vi "UpdateArrayHeightWidth.vi"(7 "Borders in Percent(T) or Pixels (F)":bool, 8 "error in (no error)":errorcluster, 9 "Adjust":u16(ring) items=["Height", "Width", "Both"], 10 "Borders":T1, 11 "Array in":refnum<vi>) -> (0 "error out":errorcluster)   [LabVIEW 2022 SP3, in "PentaPanesLibrary.lvlib" / "PentaPanes.lvclass"]
uses:
  PentaPanes.lvclass
  BordersCluster.ctl
  <vilib>/Utility/miscctls.llb/LVPositionTypeDef.ctl
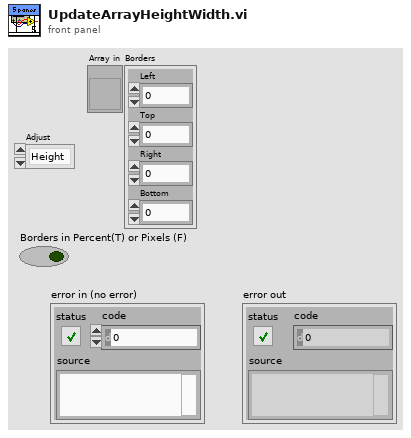
[diagram p1: front panel]
types:
  T1 = typedef "PentaPanesLibrary.lvlib/PentaPanes.lvclass/BordersCluster.ctl" = cluster{"Left":i32, "Top":i32, "Right":i32, "Bottom":i32}
  T2 = typedef "LVPositionTypeDef.ctl" = cluster{"Left":i32, "Top":i32}
  T3 = typedef "LVBoundsTypeDef.ctl" = cluster{"Width":u32, "Height":u32}
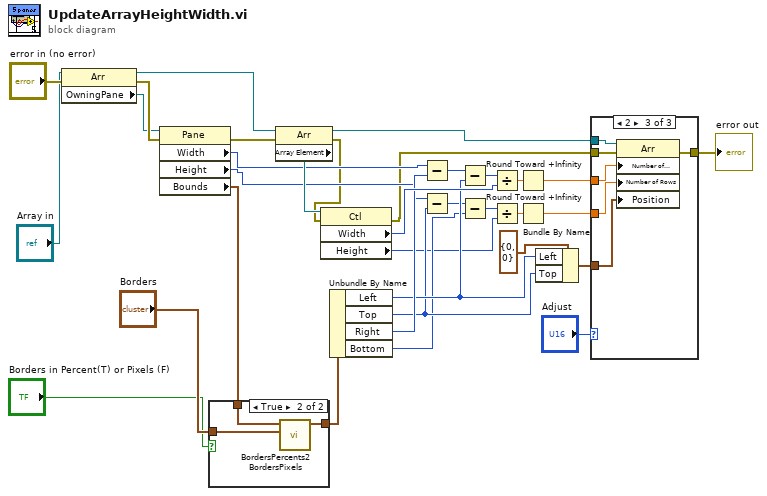
[diagram p0: block diagram]
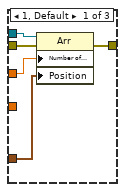
[diagram p3: hidden frame]
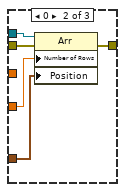
[diagram p4: hidden frame]
diagram:
  n1 = property class="Arr"(reference="Array in", error in="error in (no error)") -> (reference out=w3:refnum<vi>, error out=w33:errorcluster, "OwningPane"=w31:refnum<vi>)
  n2 = property class="Pane"(reference=w31, error in=w33) -> (error out=w7:errorcluster, "Width"=w24:u32, "Height"=w19:u32, "Bounds"=w11:T3)  [unwired: 1 out]
  n3 = case shown="True" "Borders in Percent(T) or Pixels (F)" {
    tunnel: w11 -> [_ w38]
    tunnel: "Borders" -> [w35 w37]
    tunnel: [w35 w36] -> w9
    frame False {
    }
    frame True {
      n4 = call "BordersPercents2BordersPixels.vi"("Borders in"=w37, "Bounds"=w38) -> ("Borders out"=w36:T1)  [unwired: 9 in]
    }
  }
  n5 = property class="Arr"(reference=w3, error in=w7) -> (reference out=w4:refnum<vi>, error out=w6:errorcluster, "Array Element"=w29:refnum<vi>)
  n6 = property class="Ctl"(reference=w29, error in=w6) -> (error out=w5:errorcluster, "Width"=w28:u32, "Height"=w14:u32)  [unwired: 1 out]
  n7 = Unbundle By Name(w9) -> ("Left"=w21:i32, "Top"=w18:i32, "Right"=w23:i32, "Bottom"=w16:i32)
  n8 = Subtract(x=w24, y=w23) -> (x-y=w22:u32)
  n9 = Subtract(x=w19, y=w18) -> (x-y=w17:u32)
  n10 = Subtract(x=w22, y=w21) -> (x-y=w20:u32)
  n11 = Subtract(x=w17, y=w16) -> (x-y=w15:u32)
  n12 = Divide(x=w20, y=w28) -> (x/y=w30:dbl)
  n13 = Divide(x=w15, y=w14) -> (x/y=w13:dbl)
  n14 = Round Toward +Infinity(x=w30) -> (ceil(x): smallest int >= x=w1:dbl)
  n15 = Round Toward +Infinity(x=w13) -> (ceil(x): smallest int >= x=w2:dbl)
  n16 = Bundle By Name(cluster=T2 {"Left"=0, "Top"=0} ("Position"), "Left"=w21, "Top"=w18) -> (w25:T2)
  n17 = case shown="2" "Adjust" {
    tunnel: w5 -> [w43 w48 w54]
    tunnel: [w42 w47 w53] -> w32
    tunnel: w1 -> [w41 _ w49]
    tunnel: w4 -> [w40 w46 w52]
    tunnel: w25 -> [w39 w45 w51]
    tunnel: w2 -> [_ w44 w50]
    frame 1, Default {
      n18 = property class="Arr"(reference=w40, error in=w43, "Number of Columns"=w41, "Position"=w39) -> (error out=w42:errorcluster)  [unwired: 1 out]
    }
    frame 0 {
      n19 = property class="Arr"(reference=w46, error in=w48, "Number of Rows"=w44, "Position"=w45) -> (error out=w47:errorcluster)  [unwired: 1 out]
    }
    frame 2 {
      n20 = property class="Arr"(reference=w52, error in=w54, "Number of Columns"=w49, "Number of Rows"=w50, "Position"=w51) -> (error out=w53:errorcluster)  [unwired: 1 out]
    }
  }
  "error out" <- w32
